vi "Driving By NavX.vi"(1 "Angle":dbl, 2 "Right Speed":dbl, 3 "Left Speed":dbl) -> ()   [LabVIEW 2018]
uses:
  <vilib>/Rock Robotics/WPI/ThirdParty/Sensors/navX/_TypeDefs/FRIC_navX_DeviceNumbersTypeDef.ctl
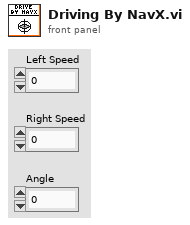
[diagram p1: front panel]
types:
  T1 = typedef "FRIC_navX_DeviceNumbersTypeDef.ctl" = enum16{"Dev0", "Dev1", "Dev2", "Dev3"}
  T2 = cluster{"Yaw":dbl, "Roll":dbl, "Pitch":dbl, "Heading":dbl, "Fused Heading":dbl}
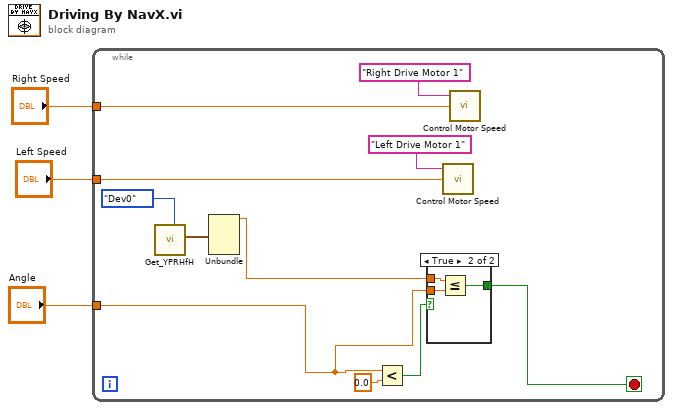
[diagram p0: block diagram]
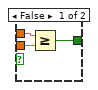
[diagram p2: hidden frame]
diagram:
  n1 = while {
    tunnel: "Angle" -> [w10]
    tunnel: "Right Speed" -> [w5]
    tunnel: "Left Speed" -> [w7]
    stop <- w9 stop-if-true
    n2 = call <vilib>:"Get_YPRHfH.vi"("Device Number"=FRIC_navX_DeviceNumbersTypeDef."Dev0") -> ("YRPHfH"=w12:T2)  [unwired: 10 in]
    n3 = Unbundle(w12) -> ("Yaw"=w11:dbl)  [unwired: 4 out]
    n4 = Less?(x=w10, y=0.0) -> (x < y?=w13:bool)
    n5 = case shown="True" w13 {
      tunnel: w10 -> [w16 w20]
      tunnel: w11 -> [w17 w19]
      tunnel: [w15 w18] -> w9
      frame False {
        n6 = Greater Or Equal?(x=w17, y=w16) -> (x >= y?=w15:bool)
      }
      frame True {
        n7 = Less Or Equal?(x=w19, y=w20) -> (x <= y?=w18:bool)
      }
    }
    n8 = call "Control Motor Speed.vi"("Speed"=w7, "Motor Name"="Left Drive Motor 1") -> ()  [unwired: 2 in]
    n9 = call "Control Motor Speed.vi"("Speed"=w5, "Motor Name"="Right Drive Motor 1") -> ()  [unwired: 2 in]
  }
